vi "Build2DArrayFromMultilineString.vi"(0 "String":string, 1 "Separator":enum16{"\\s", "\\t"}(ring)) -> (14 "2D Array out":string[][](array[string]))   [LabVIEW 2014]
doc: "This VI builds a 2D array from a multiline text string.\nAs a separator for the columns one can choose either a TAB (\\t) or a SPACE (\\s) constant.\n\nThis VI is a sub VI for the fast alignment routine managing VIs."
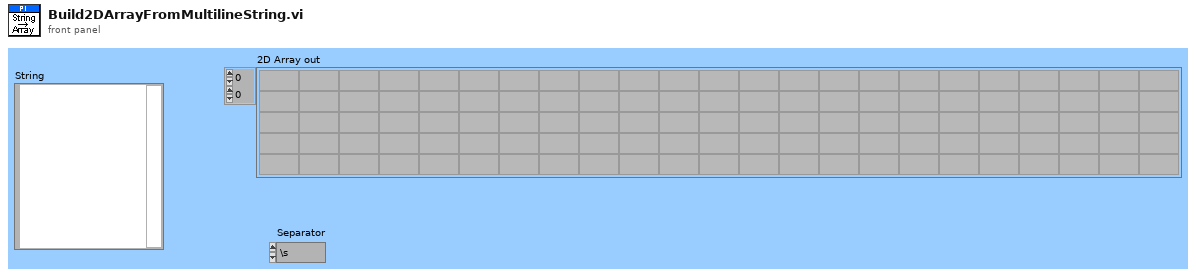
[diagram p1: front panel]
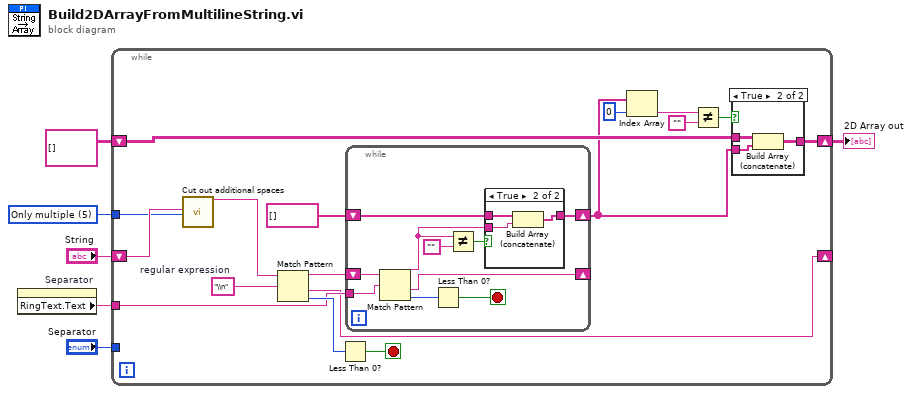
[diagram p0: block diagram]
diagram:
  w1 = u16 5 items=["All Spaces", "Only if 1st char.", "Only if last char.", "Only if near \"=\"", "Only if 1st or last char.", "Only multiple", "Really all"] ("Mode")
  n1 = property on="Separator" class="Enum (strict)"() -> ("RingText.Text"=w2:string)  [unwired: 2 in, 2 out]
  n2 = while {
    shift-right: [w17] -> _
    shift-left: "String" -> [w9]
    shift-right: [w19] -> w4
    shift-left: string[][] [] -> [w15]
    tunnel: "Separator" -> [_]
    tunnel: w2 -> [w18]
    tunnel: w1 -> [w7]
    stop <- w21 stop-if-true
    w23 = "\\n"  # regular expression
    n3 = call "Cut out additional spaces.vi"("String"=w9, "Mode"=w7) -> ("String out"=w8:string)  [unwired: 17 out]
    n4 = Match Pattern(string=w8, regular expression=w23) -> (before substring=w20:string, after substring=w17:string, offset past match=w22:i32)  [unwired: 2 out]
    n5 = Less Than 0?(x=w22) -> (x < 0?=w21:bool)
    n6 = while {
      shift-right: [w33] -> _
      shift-left: w20 -> [w37]
      shift-right: [w34] -> w14
      shift-left: string[] [] -> [w35]
      tunnel: w18 -> [w36]
      stop <- w31 stop-if-true
      n7 = Match Pattern(string=w37, regular expression=w36) -> (before substring=w30:string, after substring=w33:string, offset past match=w32:i32)  [unwired: 2 out]
      n8 = Less Than 0?(x=w32) -> (x < 0?=w31:bool)
      n9 = Not Equal?(x=w30, y="") -> (x != y?=w28:bool)
      n10 = case shown="True" w28 {
        tunnel: w35 -> [w38 w41]
        tunnel: [w38 w40] -> w34
        tunnel: w30 -> [_ w39]
        frame False {
        }
        frame True {
          n11 = Build Array (concatenate)(w41, w39) -> (w40:string[])
        }
      }
    }
    n12 = Index Array(array=w14, index=0) -> (element=w13:string)
    n13 = Not Equal?(x=w13, y="") -> (x != y?=w10:bool)
    n14 = case shown="True" w10 {
      tunnel: w15 -> [w24 w27]
      tunnel: [w24 w26] -> w19
      tunnel: w14 -> [_ w25]
      frame False {
      }
      frame True {
        n15 = Build Array (concatenate)(w27, w25) -> (w26:string[][])
      }
    }
  }
  "2D Array out" <- w4
